vi "extract FFT matrix fix I.vi"(5 "I index":i32, 7 "all field rows":dbl[][](array[numeric]), 10 "parameter":dbl[][](array[numeric]), 11 "all data rows":dbl[][](array[numeric])) -> (2 "plot parameter":T1, 3 "FFT matrix":dbl[][](array[numeric]))   [LabVIEW 2021]
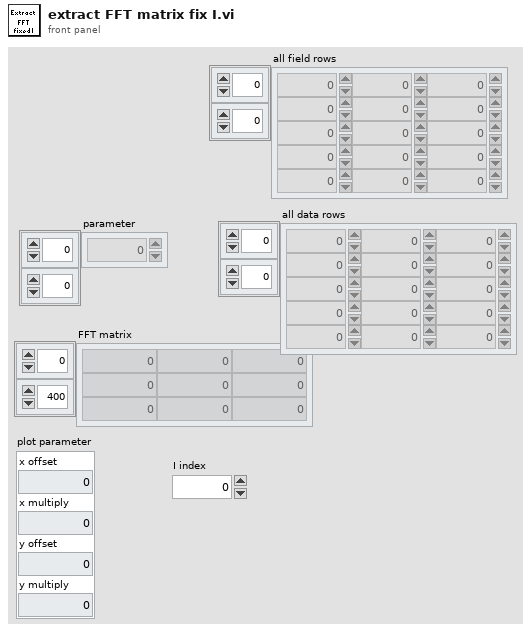
[diagram p1: front panel]
types:
  T1 = cluster{"x offset":dbl, "x multiply":dbl, "y offset":dbl, "y multiply":dbl}
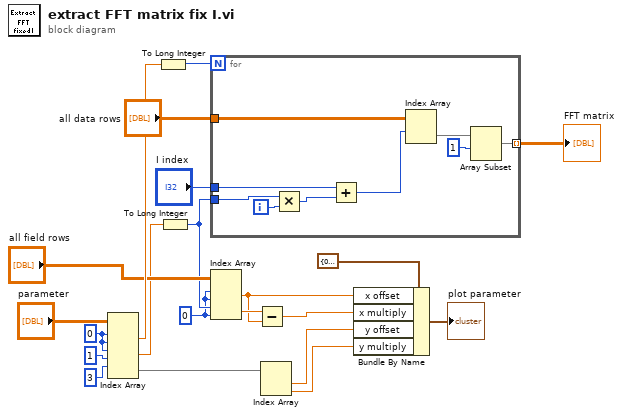
[diagram p0: block diagram]
diagram:
  w8 = 0 ("index (row)")
  w16 = 0 ("index (row)")
  n1 = Index Array(array="parameter", index (row) #1=w16, index (col) #1=w16, index (row) #2=w16, index (col) #2=1 ("disabled index (col)"), index (row) #3=3 ("index (row)")) -> (element #1=w21:dbl, element #2=w14:dbl, element #3=w3:dbl[])  [unwired: 1 in]
  n2 = To Long Integer(number=w21) -> (32bit integer=w18:i32)
  n3 = To Long Integer(number=w14) -> (32bit integer=w9:i32)
  n4 = for {
    N: w18 -> [_]
    tunnel: "all data rows" -> [w30]
    tunnel: w9 -> [w28]
    tunnel: "I index" -> [w26]
    tunnel: [w22] -> w12 mode=indexing
    i -> [w29]
    n5 = Multiply(x=w28, y=w29) -> (x*y=w27:i32)
    n6 = Add(x=w26, y=w27) -> (x+y=w25:i32)
    n7 = Index Array(array=w30, index (row)=w25) -> (element=w24:dbl[])  [unwired: 1 in]
    n8 = Array Subset(array=w24, index=1) -> (w22:dbl[])  [unwired: 1 in]
  }
  "FFT matrix" <- w12
  n9 = Index Array(array="all field rows", index (row) #1=w8, index (col) #1=w8, index (row) #2=w9, index (col) #2=w8) -> (element #1=w6:dbl, element #2=w7:dbl)
  n10 = Subtract(x=w7, y=w6) -> (x-y=w5:dbl)
  n11 = Index Array(array=w3) -> (element #1=w2:dbl, element #2=w1:dbl)  [unwired: 2 in]
  n12 = Bundle By Name(cluster=T1 {"x offset"=0.0, "x multiply"=0.0, "y offset"=0.0, "y multiply"=0.0} ("plot parameter"), "x offset"=w6, "x multiply"=w5, "y offset"=w2, "y multiply"=w1) -> (→"plot parameter":T1)
